vi "database pointer and path.vi"(6 "File Path in":path, 9 "access (0:read/write)":enum16{"read/write", "read-only", "write-only"}(ring)=enum."read-only", 10 "select source":enum32{"user selectable", "constant"}(ring), 11 "operation (0:open)":T1(ring)) -> (1 "refnum out":refnum<file>, 3 "appended path":path)   [LabVIEW 2011]
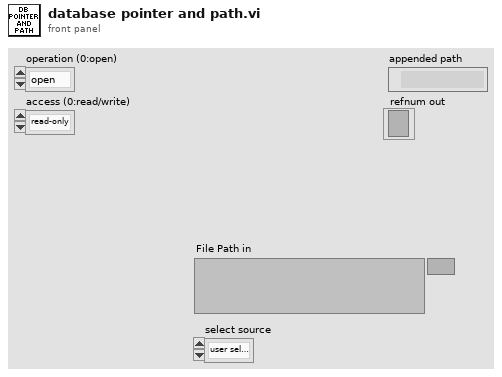
[diagram p1: front panel]
types:
  T1 = enum16{"open", "replace", "create", "open or create", "replace or create", "replace or create with confirmation"}
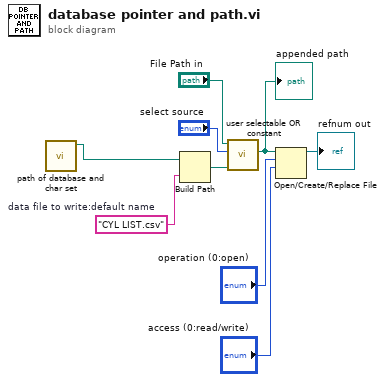
[diagram p0: block diagram]
diagram:
  w9 = "CYL LIST.csv"  # data file to write:default name
  n1 = call "path of database and char set.vi"() -> ("appended path"=w1:path)  [unwired: 11 in]
  n2 = Build Path(base path=w1, name or relative path=w9) -> (appended path=w2:path)
  n3 = call "user selectable OR constant.vi"("Constant Path in"=w2, "select source"="select source", "File Path in"="File Path in") -> ("appended path"=w3:path)  [unwired: 8 in]
  "appended path" <- w3
  n4 = Open/Create/Replace File(file path (use dialog)=w3, operation (0:open)="operation (0:open)", access (0:read/write)="access (0:read/write)") -> (refnum out=→"refnum out":refnum<file>)  [unwired: 1 in, 4 out]
